vi "Material-ConfigPage-GetEventRegistrations.vi"(11 "Configuration Page":refnum<class "Material-ConfigPage.lvclass">) -> (0 "Events":T1, 3 "Configuration Page out":refnum<class "Material-ConfigPage.lvclass">)   [LabVIEW 2013, in "Material-ConfigPage.lvclass"]
uses:
  Material-ConfigPage.lvclass
  Reuse Library/featherweight/Core/Messaging/Message/FTW-Message.lvclass
  Material-ConfigPage.lvclass/Material-ConfigPage.ctl
panel:
  # "Inputs"
  # "Outputs"
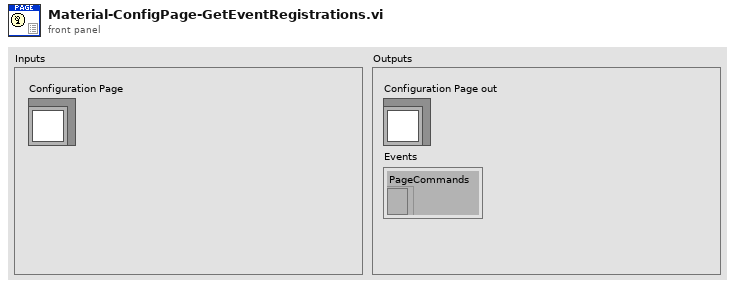
[diagram p1: front panel]
types:
  T1 = cluster{"PageCommands":refnum<event-registration>}
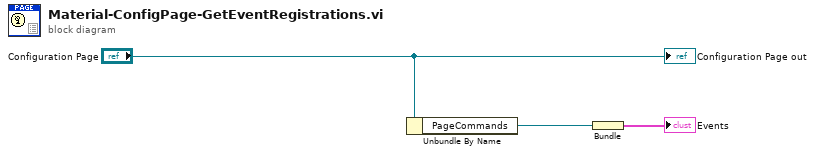
[diagram p0: block diagram]
diagram:
  n1 = Unbundle By Name("Configuration Page") -> ("PageCommands"=w2:refnum<event-registration>)
  n2 = Bundle("PageCommands"=w2) -> (→"Events":T1)  [unwired: 1 in]
  "Configuration Page out" <- "Configuration Page"
